vi "_get Session Name for PN.vi"(8 "error in (no error)":errorcluster, 11 "OBJ - Session in":refnum<class "Sequence Automation Session.lvclass">) -> (0 "error out":errorcluster, 2 "Session Name":string, 3 "OBJ - Session out":refnum<class "Sequence Automation Session.lvclass">)   [LabVIEW 2018, in "Sequence Automation Session.lvlib" / "Sequence Automation Session.lvclass"]
doc: "Wrapped Call to maintain reverse compatibility\nOnly difference is connector pane"
uses:
  Sequence Automation Session.lvclass
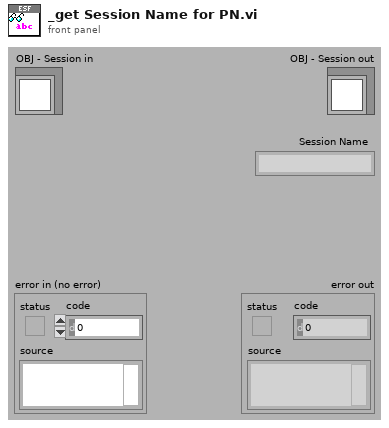
[diagram p1: front panel]
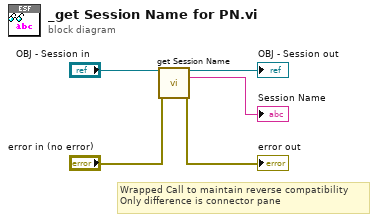
[diagram p0: block diagram]
diagram:
  # "Wrapped Call to maintain reverse compatibility\nOnly difference is connector pane"
  n1 = call "get Session Name.vi"("OBJ - Session in"="OBJ - Session in", "error in (no error)"="error in (no error)") -> ("OBJ - Session out"=→"OBJ - Session out":refnum<class "Sequence Automation Session.lvclass">, "Session Name"=→"Session Name":string, "error out"=→"error out":errorcluster)  [unwired: 11 in]
